vi "Working Shift Change(A-B &C) new.vi"(11 "input cluster":T1) -> (3 "Shift Change":string="A")   [LabVIEW 2015]
doc: "this vi only used for industial working shifting hour from A to C shift . user can be set the shift time from A to C."
panel:
  out "appended array":bool[](array[boolean])=[TRUE, FALSE, FALSE]
  out "Actual Time":i32=60000
  out "current time":timestamp=timestamp(3659733000.181 s since 1904-01-01)
  out "Shift change":u8=1
  # "145801"
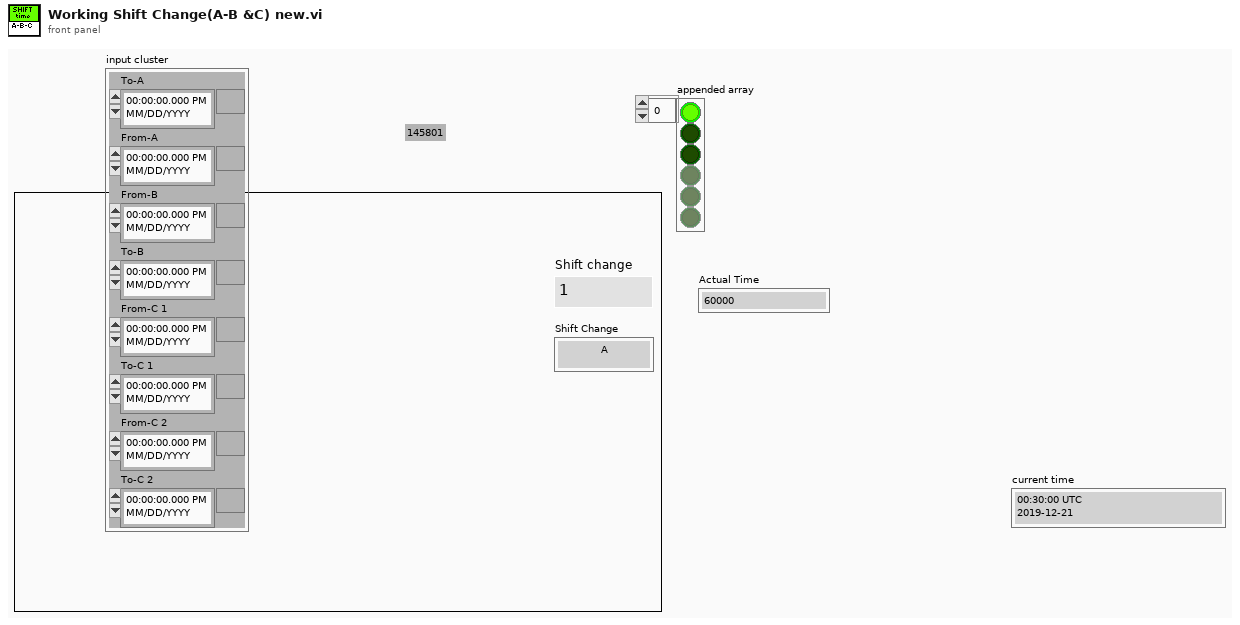
[diagram p1: front panel]
types:
  T1 = cluster{"To-A":timestamp, "From-A":timestamp, "From-B":timestamp, "To-B":timestamp, "From-C 1":timestamp, "To-C 1":timestamp, "From-C 2":timestamp, "To-C 2":timestamp}
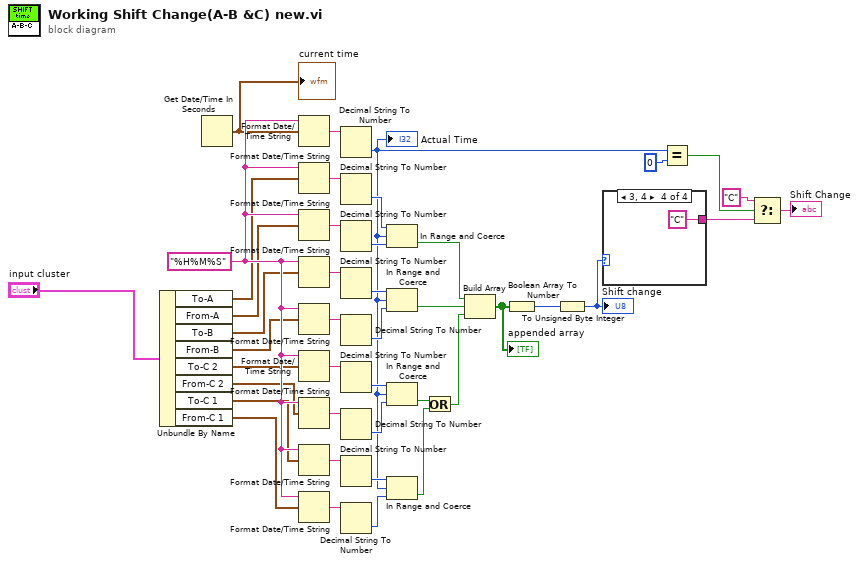
[diagram p0: block diagram]
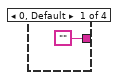
[diagram p2: hidden frame]
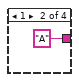
[diagram p3: hidden frame]
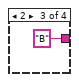
[diagram p4: hidden frame]
diagram:
  w25 = "%H%M%S" ("time format string (%c)")
  n1 = Unbundle By Name("input cluster") -> ("To-A"=w9:timestamp, "From-A"=w8:timestamp, "To-B"=w7:timestamp, "From-B"=w6:timestamp, "To-C 2"=w5:timestamp, "From-C 2"=w4:timestamp, "To-C 1"=w3:timestamp, "From-C 1"=w2:timestamp)
  n2 = Get Date/Time In Seconds() -> (seconds since 1Jan1904=w16:timestamp)
  "current time" <- w16
  n3 = Format Date/Time String(time format string (%c)=w25, seconds (now)=w16) -> (date/time string=w41:string)  [unwired: 1 in]
  n4 = Format Date/Time String(time format string (%c)=w25, seconds (now)=w9) -> (date/time string=w40:string)  [unwired: 1 in]
  n5 = Format Date/Time String(time format string (%c)=w25, seconds (now)=w8) -> (date/time string=w42:string)  [unwired: 1 in]
  n6 = Format Date/Time String(time format string (%c)=w25, seconds (now)=w7) -> (date/time string=w39:string)  [unwired: 1 in]
  n7 = Format Date/Time String(time format string (%c)=w25, seconds (now)=w6) -> (date/time string=w38:string)  [unwired: 1 in]
  n8 = Format Date/Time String(time format string (%c)=w25, seconds (now)=w5) -> (date/time string=w35:string)  [unwired: 1 in]
  n9 = Format Date/Time String(time format string (%c)=w25, seconds (now)=w4) -> (date/time string=w36:string)  [unwired: 1 in]
  n10 = Format Date/Time String(time format string (%c)=w25, seconds (now)=w3) -> (date/time string=w26:string)  [unwired: 1 in]
  n11 = Format Date/Time String(time format string (%c)=w25, seconds (now)=w2) -> (date/time string=w27:string)  [unwired: 1 in]
  n12 = Decimal String To Number(string=w41) -> (number=w15:i32)  [unwired: 2 in, 1 out]
  "Actual Time" <- w15
  n13 = Decimal String To Number(string=w40) -> (number=w29:i32)  [unwired: 2 in, 1 out]
  n14 = Decimal String To Number(string=w42) -> (number=w28:i32)  [unwired: 2 in, 1 out]
  n15 = Decimal String To Number(string=w39) -> (number=w17:i32)  [unwired: 2 in, 1 out]
  n16 = Decimal String To Number(string=w38) -> (number=w37:i32)  [unwired: 2 in, 1 out]
  n17 = Decimal String To Number(string=w35) -> (number=w21:i32)  [unwired: 2 in, 1 out]
  n18 = Decimal String To Number(string=w36) -> (number=w22:i32)  [unwired: 2 in, 1 out]
  n19 = Decimal String To Number(string=w26) -> (number=w24:i32)  [unwired: 2 in, 1 out]
  n20 = Decimal String To Number(string=w27) -> (number=w23:i32)  [unwired: 2 in, 1 out]
  n21 = In Range and Coerce(upper limit=w29, x=w15, lower limit=w28) -> (In Range?=w34:bool)  [unwired: 1 out]
  n22 = In Range and Coerce(upper limit=w17, x=w15, lower limit=w37) -> (In Range?=w33:bool)  [unwired: 1 out]
  n23 = In Range and Coerce(upper limit=w21, x=w15, lower limit=w22) -> (In Range?=w20:bool)  [unwired: 1 out]
  n24 = In Range and Coerce(upper limit=w24, x=w15, lower limit=w23) -> (In Range?=w19:bool)  [unwired: 1 out]
  n25 = Or(x=w20, y=w19) -> (x .or. y?=w18:bool)
  n26 = Build Array(w34, w33, w18) -> (w32:bool[])
  "appended array" <- w32
  n27 = Boolean Array To Number(Boolean array=w32) -> (number=w31:u32)
  n28 = To Unsigned Byte Integer(number=w31) -> (unsigned 8bit integer=w30:u8)
  "Shift change" <- w30
  n29 = case shown="3, 4" w30 {
    tunnel: ["" "A" "B" "C"] -> w11
    frame 0, Default {
    }
    frame 1 {
    }
    frame 2 {
    }
    frame 3, 4 {
    }
  }
  n30 = Equal?(x=w15, y=0) -> (x = y?=w13:bool)
  n31 = Select(t="C", s=w13, f=w11) -> (s? t:f=→"Shift Change":string)
